vi "OCR_OCR MAIN.vi"(8 "Error":errorcluster, 11 "ICON Cluster":T1={"Header"="", "Body"=[], "ImageData"={"image type"=0, "image depth"=0, "image"=[], "mask"=[], "colors"=[], "Rectangle"={"left"=0, "top"=0, "right"=0, "bottom"=0}}, "New Icon"=bytes[0], "Line Status"=[], "Format"={"Color"={"Body txt"=255, "Body Back"=12632256, "Frame"=0, "Header txt"=32768, "Header Back"=16744703, "type"=enum."2 Color"}, "Icon Sizing"={"Rule"=enum."Static", "Header"=TRUE, "Rows"=5, "Width"=32, "Position"=enum."MID-CTR"}}} {"Format"."Icon Sizing"."Rows" min=1 max=5 step=1; "Format"."Icon Sizing"."Width" min=7 max=32 step=1}) -> (0 "Error Out":errorcluster, 3 "ICON Cluster Out":T1={"Header"="", "Body"=[], "ImageData"={"image type"=0, "image depth"=0, "image"=[], "mask"=[], "colors"=[], "Rectangle"={"left"=0, "top"=0, "right"=0, "bottom"=0}}, "New Icon"=bytes[0], "Line Status"=[], "Format"={"Color"={"Body txt"=255, "Body Back"=12632256, "Frame"=0, "Header txt"=32768, "Header Back"=16744703, "type"=enum."2 Color"}, "Icon Sizing"={"Rule"=enum."Static", "Header"=TRUE, "Rows"=5, "Width"=32, "Position"=enum."MID-CTR"}}} {"Format"."Icon Sizing"."Rows" min=1 max=5 step=1; "Format"."Icon Sizing"."Width" min=7 max=32 step=1})   [LabVIEW 2009]
doc: "Fills in the text and color data using the Image Data"
uses:
  Controls/Cluster/Cluster_Icon Data.ctl
  Controls/String_Picture/STRING_Line Display.ctl
  Controls/Array/String Array_Body Text.ctl
  Controls/Cluster/Cluster_Image Data.ctl
  Controls/Cluster/CLuster_Selectoin Box.ctl
  Controls/String_Picture/Picture_Icon.ctl
  Controls/Cluster/Cluster_Icon Format.ctl
  Controls/Cluster/Cluster_Icon Color Set.ctl
  Controls/Enum/ENUM_Frame Template Select.ctl
  Controls/Cluster/Cluster_Sizing Data.ctl
  Controls/Enum/ENUM_Icon Sizing.ctl
  Controls/Enum/RBENUM_Icon Position.ctl
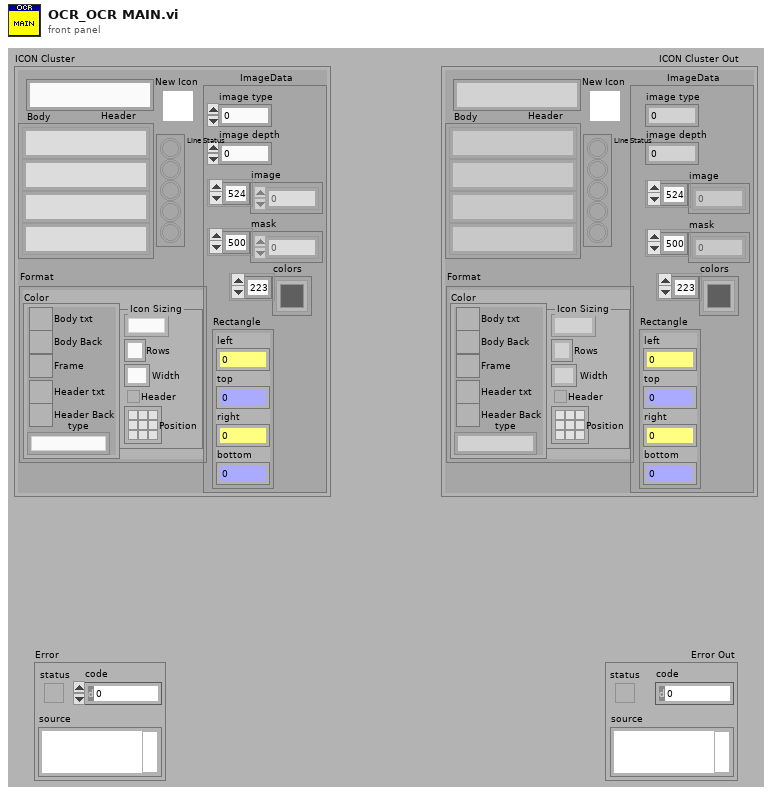
[diagram p1: front panel]
types:
  T1 = typedef "Cluster_Icon Data.ctl" = cluster{"Header":T2, "Body":T3, "ImageData":T4, "New Icon":T6, "Line Status":bool[], "Format":T7}
  T2 = typedef "STRING_Line Display.ctl" = string
  T3 = typedef "String Array_Body Text.ctl" = T2[]
  T4 = typedef "Cluster_Image Data.ctl" = cluster{"image type":i32, "image depth":i32, "image":u8[], "mask":u8[], "colors":u32[], "Rectangle":T5}
  T5 = typedef "CLuster_Selectoin Box.ctl" = cluster{"left":i16, "top":i16, "right":i16, "bottom":i16}
  T6 = typedef "Picture_Icon.ctl" = picture
  T7 = typedef "Cluster_Icon Format.ctl" = cluster{"Color":T8, "Icon Sizing":T10}
  T8 = typedef "Cluster_Icon Color Set.ctl" = cluster{"Body txt":u32, "Body Back":u32, "Frame":u32, "Header txt":u32, "Header Back":u32, "type":T9}
  T9 = typedef "ENUM_Frame Template Select.ctl" = enum16{"2 Color", "5 Color"}
  T10 = typedef "Cluster_Sizing Data.ctl" = cluster{"Rule":T11, "Header":bool, "Rows":u32, "Width":u32, "Position":T12}
  T11 = typedef "ENUM_Icon Sizing.ctl" = enum16{"Static", "Auto"}
  T12 = typedef "RBENUM_Icon Position.ctl" = enum32{"LFT-TOP", "MID-TOP", "RGT-TOP", "LFT-CTR", "MID-CTR", "RGT-CTR", "LFT-BOT", "MID-BOT", "RGT-BOT"}
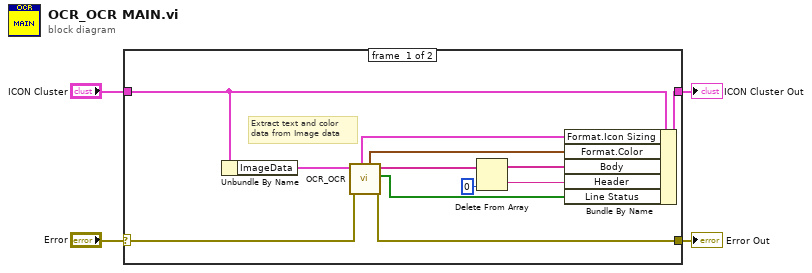
[diagram p0: block diagram]
diagram:
  n1 = case shown="No Error" "Error" {
    selector: "Error" -> [w15 w18]
    tunnel: "ICON Cluster" -> [w9 w17]
    tunnel: [w16 w17] -> w2
    tunnel: [w14 w18] -> w1
    frame #0 {
      # "Extract text and color\ndata from Image data"
      n2 = Unbundle By Name(w9) -> ("ImageData"=w10:T4)
      n3 = call "OCR_OCR.vi"("Error"=w15, "Image Data"=w10) -> ("Error Out"=w14:errorcluster, "Status Of Each Line Out"=w6:bool[], "Text Out"=w13:T2[], "Colors Out"=w8:T8, "Icon Sizing Out"=w7:T10)  [unwired: 5 in]
      n4 = Delete From Array(array=w13, index=0) -> (deleted portion=w12:T2, array with subset deleted=w11:T2[])  [unwired: 1 in]
      n5 = Bundle By Name(cluster=w9, "Format.Icon Sizing"=w7, "Format.Color"=w8, "Body"=w11, "Header"=w12, "Line Status"=w6) -> (w16:T1)
    }
    frame #1 {
    }
  }
  "Error Out" <- w1
  "ICON Cluster Out" <- w2
